vi "test-PLT-2.vi"() -> ()   [LabVIEW 2014]
doc: "André Romero - 2016\nandretec@ifsc.usp.br"
panel:
  in  "Density":dbl=10.0
  in  "Scale":dbl=5.0
  in  "Scale by":enum16{"X", "Y", "XY"}(ring)=enum."Y"
  out "XY Graph 2":cluster{"X out":dbl[], "Y out":dbl[]}(graph)
  out "XY Graph":cluster{"Array":ext[], "Array 2":ext[]}(graph)={"Array"=[-796.5, -1072.5, -1318.5, -1318.5, -678.5, -733.5, -773.5, -827.5, -869.5, -925.5, -1694.5, -1763.5, -1832.5, -1891.5, -1913.5, -1927.5, -1940.5, -1945.5, -1944.5, -1947.5, -1946.5, -1941.5, -1318.5, -1318.5, 73.5, 554.5, 571.5, 576.5, 564.5, 550.5, 521.5, 475.5, 412.5, -241.5, -352.5, -458.5, -527.5, -577.5, -622.5, -678.5, -678.5, 618.5, 568.5, 525.5, 478.5, 415.5, 263.5, 13.5, -427.5, -484.5, -545.5, -599.5, -633.5, -644.5, -648.5, -647.5, -648.5, -643.5, -630.5, -156.5, 1289.5, 1289.5, 612.5, 618.5, 661.5, 689.5, 744.5, 801.5, 864.5, 937.5, 1594.5, 1688.5, 1777.5, 1817.5, 1853.5, 1885.5, 1911.5, 1937.5, 1947.5, 1946.5, 1946.5, 1637.5, 1289.5, 693.5], "Array 2"=[735.0, 737.0, 731.0, 176.0, -599.0, -635.0, -677.0, -711.0, -721.0, -725.0, -725.0, -717.0, -694.0, -654.0, -627.0, -596.0, -536.0, -471.0, -339.0, -67.0, 93.0, 176.0, 176.0, -285.0, 318.0, -163.0, -255.0, -375.0, -596.0, -658.0, -701.0, -727.0, -735.0, -735.0, -737.0, -730.0, -705.0, -670.0, -632.0, -599.0, -308.0, 576.0, 612.0, 653.0, 689.0, 711.0, 718.0, 719.0, 715.0, 705.0, 679.0, 640.0, 593.0, 547.0, 492.0, 383.0, 273.0, 222.0, 169.0, -295.0, 328.0, -721.0, 366.0, 576.0, 601.0, 637.0, 683.0, 707.0, 716.0, 718.0, 718.0, 717.0, 707.0, 693.0, 672.0, 641.0, 599.0, 524.0, 443.0, 271.0, -718.0, -724.0, -721.0, -721.0]}
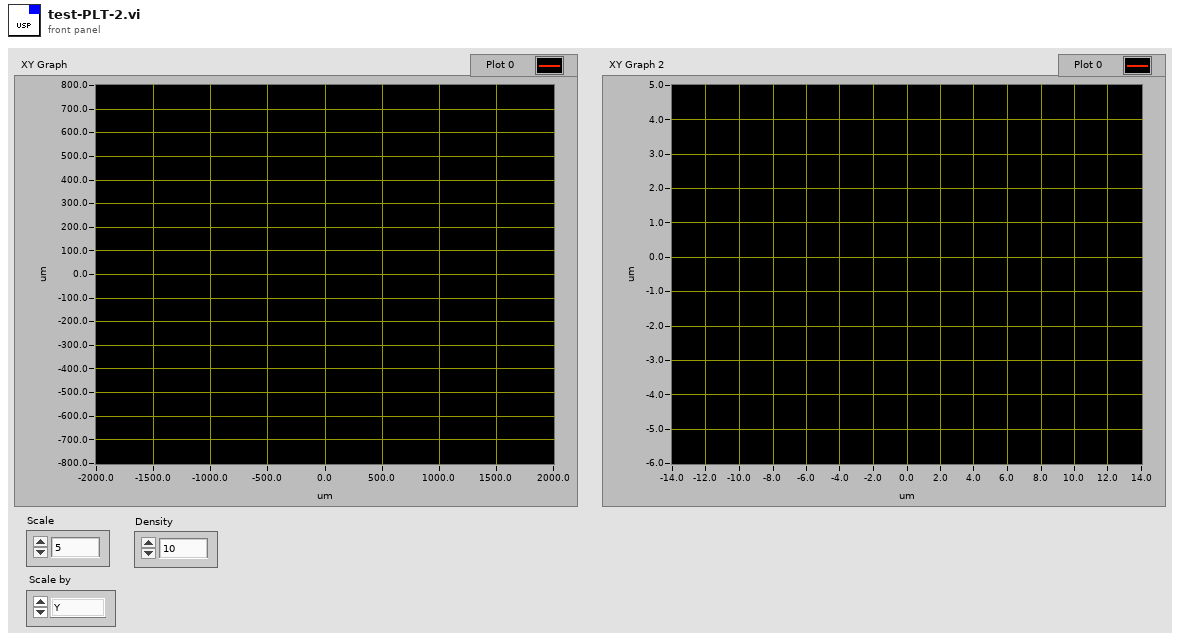
[diagram p1: front panel]
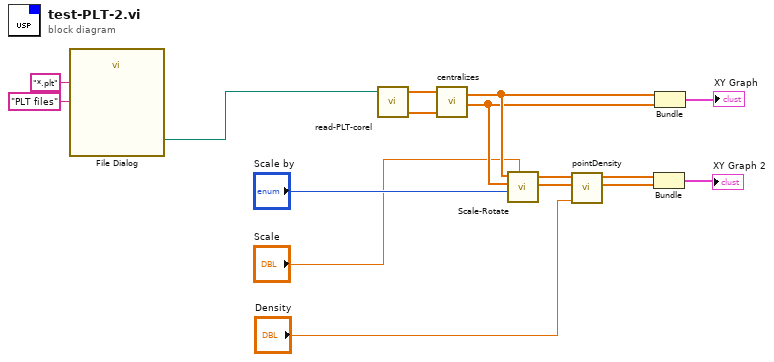
[diagram p0: block diagram]
diagram:
  n1 = call "File Dialog"("pattern (all files)"="*.plt", "pattern label"="PLT files") -> ("selected path"=w3:path)  [unwired: 10 in, 3 out]
  n2 = call "read-PLT-corel.vi"("file (use dialog)"=w3) -> ("Y"=w15:ext[], "X"=w16:ext[])  [unwired: 2 in, 1 out]
  n3 = call "centralizes.vi"("Y in"=w15, "X in"=w16) -> ("Y out"=w11:ext[], "X out"=w12:ext[])  [unwired: 2 in]
  n4 = call "Scale-Rotate.vi"("Scale"="Scale", "Scale by"="Scale by", "Y in"=w11, "X in"=w12) -> ("Y out"=w7:dbl[], "X out"=w8:dbl[])  [unwired: 6 in]
  n5 = call "pointDensity.vi"("Density"="Density", "Y in"=w7, "X in"=w8) -> ("Y out"=w4:dbl[], "X out"=w5:dbl[])  [unwired: 6 in, 1 out]
  n6 = Bundle("X out"=w5, "Y out"=w4) -> (→"XY Graph 2":cluster{"X out":dbl[], "Y out":dbl[]})  [unwired: 1 in]
  n7 = Bundle("X out"=w12, "Y out"=w11) -> (→"XY Graph":cluster{"X out":ext[], "Y out":ext[]})  [unwired: 1 in]
